vi "mb module version constant.vi"() -> (3 "current version":string="1.0.0.0")   [LabVIEW 2013, in "Modbus Slave configuration.lvclass"]
uses:
  Modbus Slave configuration.lvclass
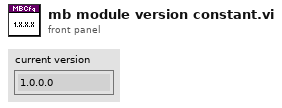
[diagram p1: front panel]
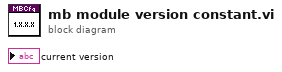
[diagram p0: block diagram]
diagram:
